vi "Process Live Data Q.vi"(8 "error in (no error)":errorcluster, 10 "Live Data Q Elements":cluster{"NI Data Waveforms":waveform(dbl)[]}[](array[cluster]), 11 "NI Force Task in":refnum<class "NI Force Task.lvclass">) -> (0 "error out":errorcluster, 3 "NI Force Task out":refnum<class "NI Force Task.lvclass">)   [LabVIEW 2020, in "NI Force Task.lvlib" / "NI Force Task.lvclass"]
uses:
  NI Force Task.lvclass
  NI Force Task.lvclass/NI Force Task.ctl
  <vilib>/Analysis/baseanly.llb/Mean (DBL).vi
  <vilib>/Analysis/NI_AALBase.lvlib
  Task Viewer Messages/Receive Q Msg/Receive Q Msg.lvclass
  Lissajous Viewer Messages/Update graph Msg/Update graph Msg.lvclass
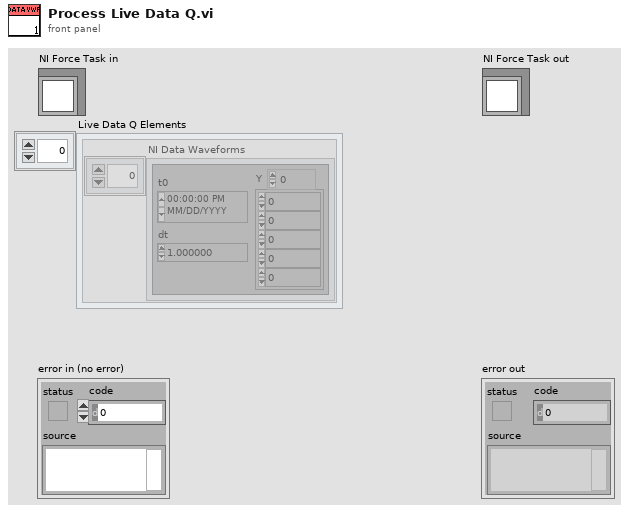
[diagram p1: front panel]
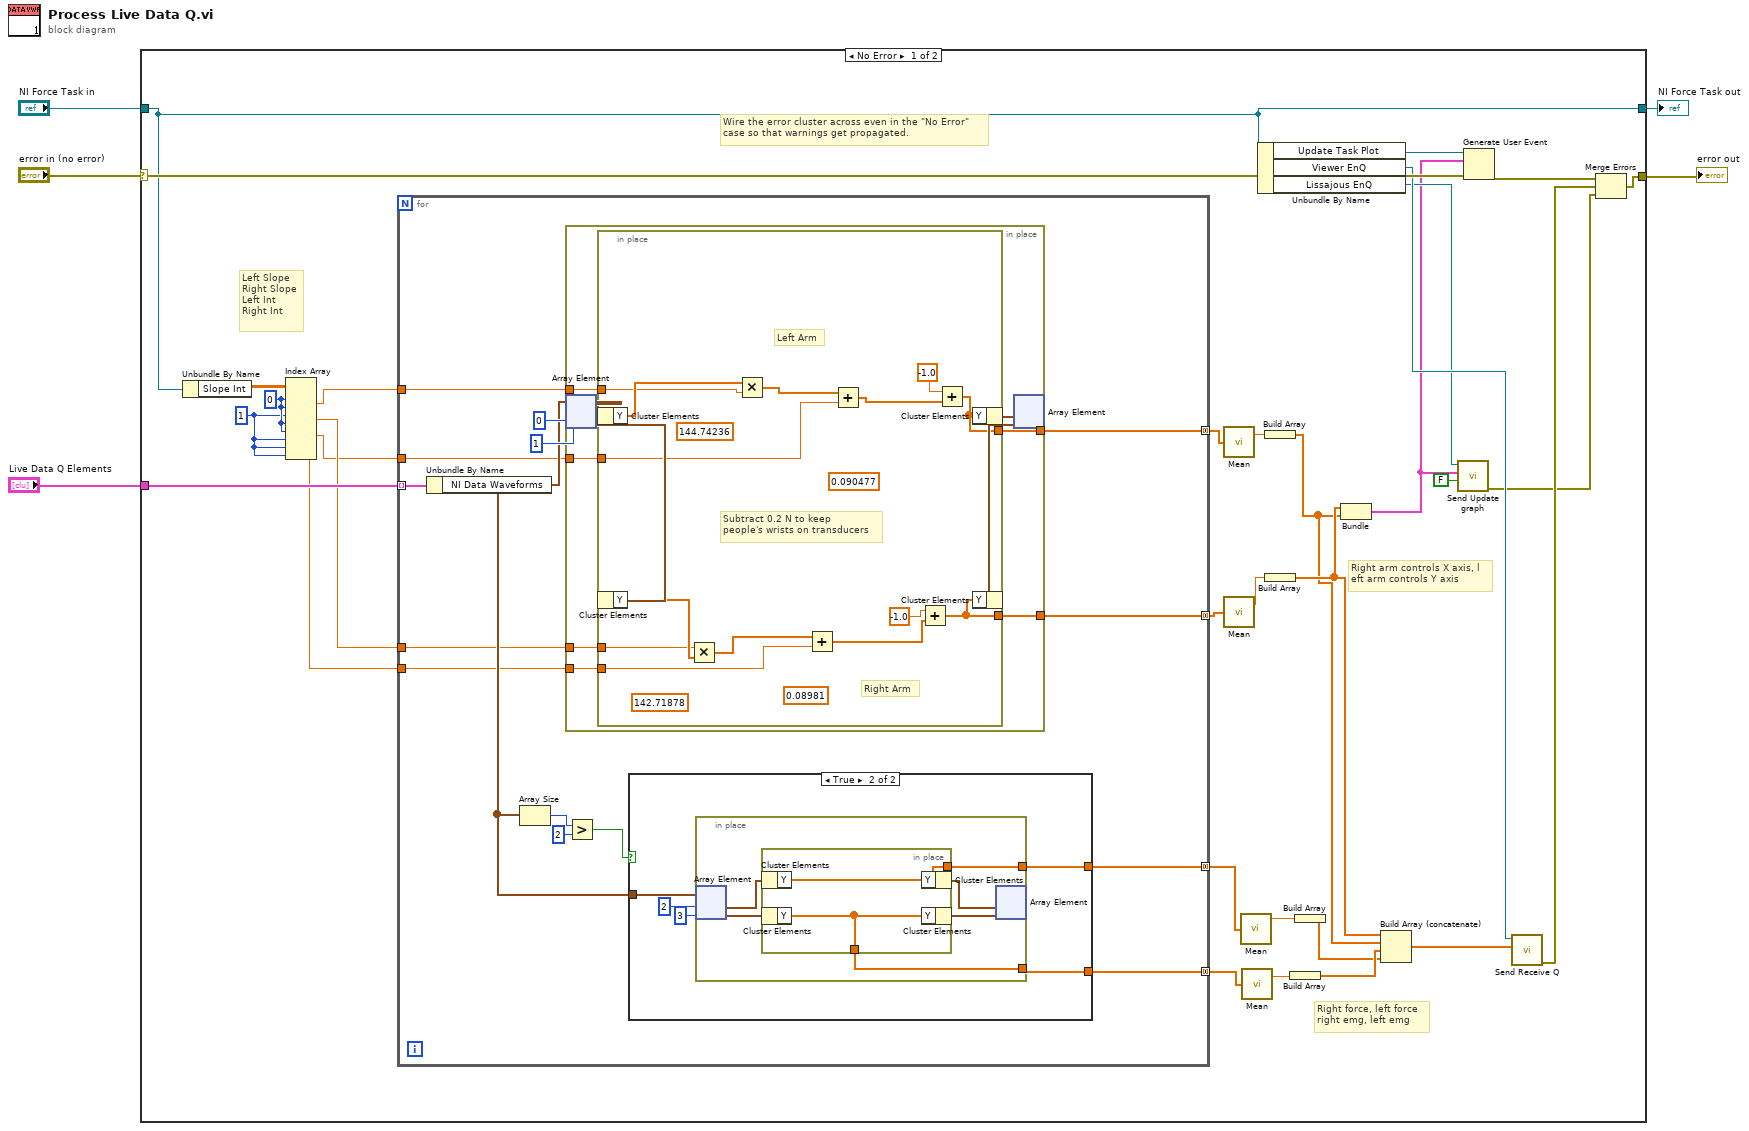
[diagram p0: block diagram]
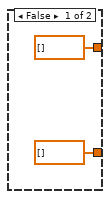
[diagram p2: hidden frame]
diagram:
  n1 = case shown="No Error" "error in (no error)" {
    selector: "error in (no error)" -> [w31 w92]
    tunnel: [w13 w93] -> w3
    tunnel: "NI Force Task in" -> [w13 w93]
    tunnel: "Live Data Q Elements" -> [w37 _]
    tunnel: [w23 w92] -> w1
    frame No Error {
      w10 = 1 ("disabled index (row)")
      w11 = 0 ("index (row)")
      # "Left Slope\nRight Slope\nLeft Int\nRight Int"
      # "Right force, left force\nright emg, left emg"
      # "Right arm controls X axis, l\neft arm controls Y axis"
      # "Wire the error cluster across even in the \"No Error\"\ncase so that warnings get propagated."
      n2 = Unbundle By Name(w13) -> ("Slope Int"=w12:dbl[][])
      n3 = Index Array(array=w12, index (row) #1=w11, index (col) #1=w11, index (row) #2=w10, index (col) #2=w11, index (row) #3=w11, index (col) #3=w10, index (row) #4=w10, index (col) #4=w10) -> (element #1=w9:dbl, element #2=w8:dbl, element #3=w7:dbl, element #4=w6:dbl)
      n4 = for {
        tunnel: w37 -> [w52] mode=indexing
        tunnel: [w50] -> w34 mode=concatenating
        tunnel: [w49] -> w33 mode=concatenating
        tunnel: [w43] -> w30 mode=concatenating
        tunnel: [w42] -> w29 mode=concatenating
        tunnel: w9 -> [w41]
        tunnel: w8 -> [w40]
        tunnel: w7 -> [w39]
        tunnel: w6 -> [w38]
        n5 = Unbundle By Name(w52) -> ("NI Data Waveforms"=w44:waveform(dbl)[])
        n6 = Array Size(array=w44) -> (size(s)=w47:i32)
        n7 = in-place {
          in-place-border: [w75] -> w50
          in-place-border: [w74] -> w49
          in-place-border: w41 -> [w71]
          in-place-border: w40 -> [w70]
          in-place-border: w39 -> [w69]
          in-place-border: w38 -> [w68]
          n8 = in-place-array #1(w44, 0, 1) -> (w77:waveform(dbl), w73:waveform(dbl))
          n9 = in-place {
            in-place-border: [w86] -> w75
            in-place-border: [w84] -> w74
            in-place-border: w71 -> [w81]
            in-place-border: w70 -> [w80]
            in-place-border: w69 -> [w79]
            in-place-border: w68 -> [w78]
            (unwired) 0.08981
            (unwired) 0.090477
            (unwired) 144.74236
            (unwired) 142.71878
            # "Left Arm"
            # "Right Arm"
            # "Subtract 0.2 N to keep \npeople's wrists on transducers"
            n10 = in-place-cluster #2(w77) -> ("Y"=w88:dbl[])
            n11 = in-place-cluster #3(w73) -> ("Y"=w89:dbl[])
            n12 = Multiply(x=w80, y=w89) -> (x*y=w90:dbl[])
            n13 = Multiply(x=w88, y=w81) -> (x*y=w91:dbl[])
            n14 = Add(x=w90, y=w78) -> (x+y=w85:dbl[])
            n15 = Add(x=w91, y=w79) -> (x+y=w87:dbl[])
            n16 = Add(x=-1.0, y=w85) -> (x+y=w84:dbl[])
            n17 = Add(x=-1.0, y=w87) -> (x+y=w86:dbl[])
            n18 = in-place-cluster #2("Y"=w86) -> (w76:waveform(dbl))
            n19 = in-place-cluster #3("Y"=w84) -> (w72:waveform(dbl))
          }
          n20 = in-place-array #1(w76, w72) -> ()  [unwired: 3 out]
        }
        n21 = Greater?(x=w47, y=2) -> (0:w45:bool)
        n22 = case shown="True" w45 {
          tunnel: w44 -> [_ w59]
          tunnel: [dbl[] [] ("Y") w56] -> w43
          tunnel: [dbl[] [] ("Y") w55] -> w42
          frame False {
          }
          frame True {
            n23 = in-place {
              in-place-border: [w61] -> w56
              in-place-border: [w60] -> w55
              n24 = in-place-array #4(w59, 2, 3) -> (w65:waveform(dbl), w64:waveform(dbl))
              n25 = in-place {
                in-place-border: [w67] -> w61
                in-place-border: [w66] -> w60
                n26 = in-place-cluster #5(w65) -> ("Y"=w67:dbl[])
                n27 = in-place-cluster #6(w64) -> ("Y"=w66:dbl[])
                n28 = in-place-cluster #5("Y"=w67) -> (w63:waveform(dbl))
                n29 = in-place-cluster #6("Y"=w66) -> (w62:waveform(dbl))
              }
              n30 = in-place-array #4(w63, w62) -> ()  [unwired: 3 out]
            }
          }
        }
      }
      n31 = call-poly <vilib>:"Mean.vi"("X"=w34) -> ("mean"=w36:dbl)  [unwired: 1 out]
      n32 = call-poly <vilib>:"Mean.vi"("X"=w33) -> ("mean"=w35:dbl)  [unwired: 1 out]
      n33 = call-poly <vilib>:"Mean.vi"("X"=w30) -> ("mean"=w27:dbl)  [unwired: 1 out]
      n34 = call-poly <vilib>:"Mean.vi"("X"=w29) -> ("mean"=w28:dbl)  [unwired: 1 out]
      n35 = Unbundle By Name(w13) -> ("Update Task Plot"=w32:refnum<user-event>, "Viewer EnQ"=w24:refnum<class "Message Enqueuer.lvclass">, "Lissajous EnQ"=w17:refnum<class "Message Enqueuer.lvclass">)
      n36 = Build Array(w36) -> (w18:dbl[])
      n37 = Build Array(w35) -> (w19:dbl[])
      n38 = Build Array(w28) -> (w26:dbl[])
      n39 = Build Array(w27) -> (w25:dbl[])
      n40 = Bundle(w19, w18) -> (w16:cluster{dbl[], dbl[]})  [unwired: 1 in]
      n41 = Build Array (concatenate)(w19, w18, w26, w25) -> (w20:dbl[])
      n42 = call "Send Update graph.vi"("Template?"=FALSE, "Data"=w16, "Message Enqueuer in"=w17) -> ("error out"=w14:errorcluster)  [unwired: 7 in, 1 out]
      n43 = Generate User Event(user event=w32, event data cluster=w16, error in=w31) -> (error out=w22:errorcluster)  [unwired: 1 in, 1 out]
      n44 = call "Send Receive Q.vi"("Disp Data"=w20, "Message Enqueuer in"=w24) -> ("error out"=w21:errorcluster)  [unwired: 8 in, 1 out]
      n45 = Merge Errors(w22, w21, w14) -> (w23:errorcluster)
    }
    frame Error {
    }
  }
  "error out" <- w1
  "NI Force Task out" <- w3
